vi "New motor Control integrated, NavX correction.vi"(1 "wTargetSpeed":dbl, 2 "yTargetSpeed":dbl, 3 "xTargetSpeed":dbl) -> (0 "Speed":T2)   [LabVIEW 2018]
panel:
  in  "Reset Encoder 0":bool
  in  "Boolean":bool=TRUE
  out "Distance":T1
  out "wSpeed":dbl
  out "ySpeed":dbl
  out "xSpeed":dbl
  out "Distance M2":dbl
  out "Distance M1":dbl
  out "Distance M0":dbl
  out "Motor Error":errorcluster
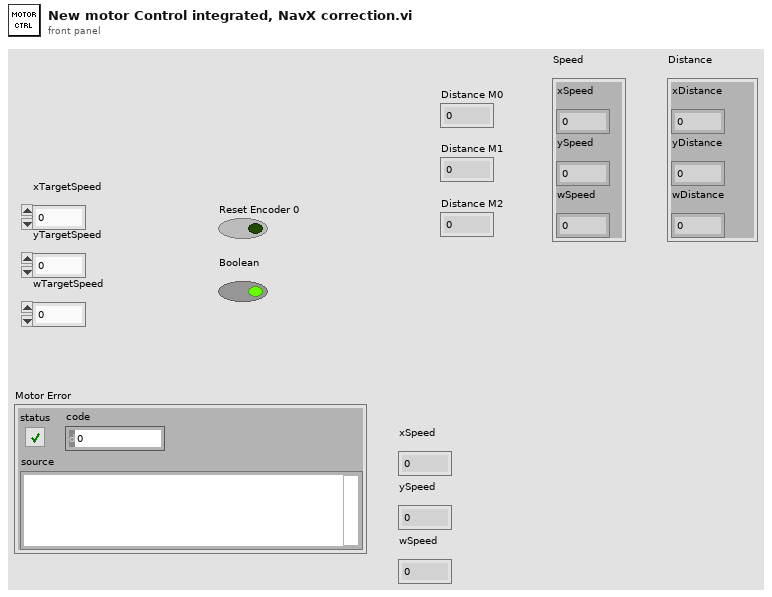
[diagram p1: front panel]
types:
  T1 = cluster{"xDistance":dbl, "yDistance":dbl, "wDistance":dbl}
  T2 = cluster{"xSpeed":dbl, "ySpeed":dbl, "wSpeed":dbl}
  T3 = cluster{"Encoder 0":dbl, "Encoder 1":dbl, "Encoder 2":dbl}
  T4 = cluster{"Distance M0 ":dbl, "Distance M1 ":dbl, "Distance M2 ":dbl}
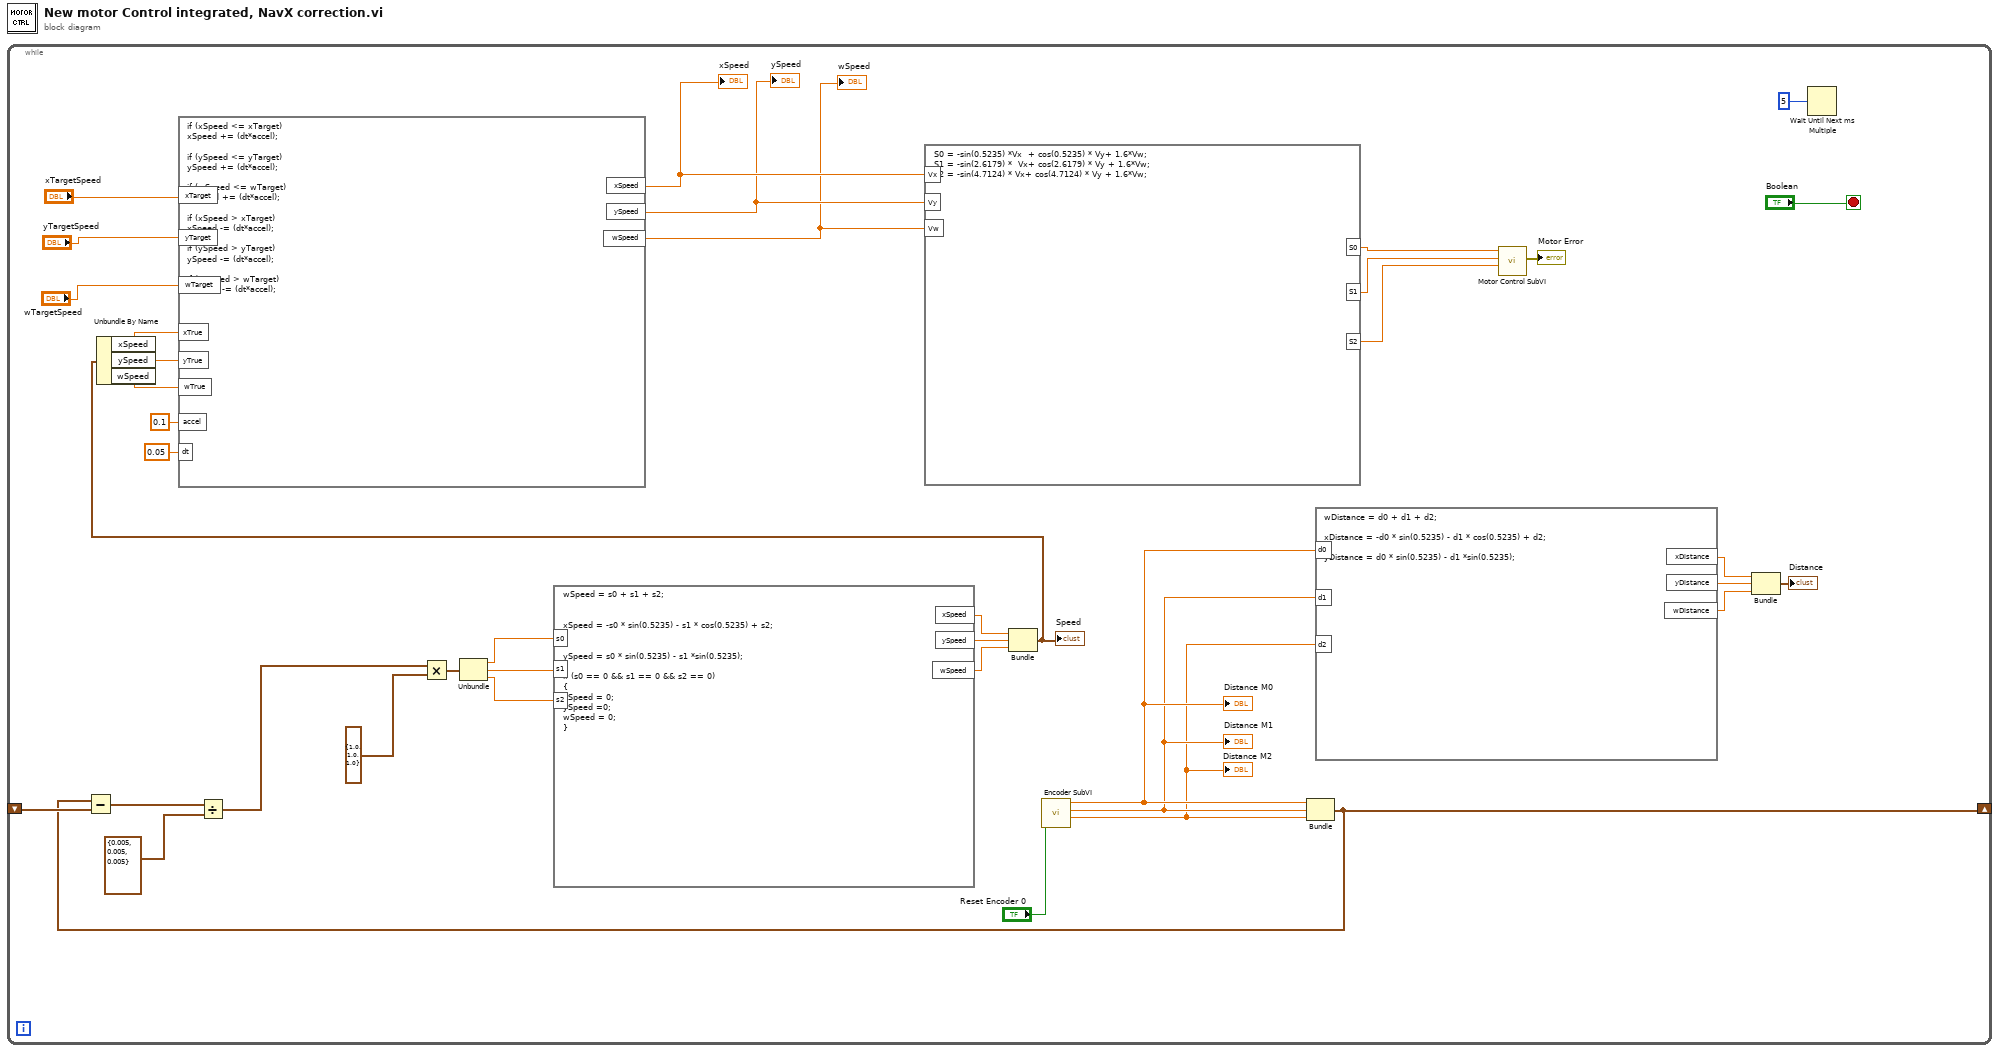
[diagram p0: block diagram]
diagram:
  n1 = while {
    shift-right: [w15] -> _
    shift-left: _ -> [w16]
    stop <- "Boolean" stop-if-true
    n2 = call "Encoder SubVI.vi"("Reset Encoders"="Reset Encoder 0") -> ("Distance M2"=w11:dbl, "Distance M1"=w12:dbl, "Distance M0"=w13:dbl)  [unwired: 7 in, 1 out]
    "Distance M0" <- w13
    "Distance M1" <- w12
    "Distance M2" <- w11
    n3 = Bundle("Distance M0"=w13, "Distance M1"=w12, "Distance M2"=w11) -> (w15:T4)  [unwired: 1 in]
    n4 = Subtract(x=w15, y=w16) -> (x-y=w38:T4)
    n5 = Divide(x=w38, y=T3 {"Encoder 0"=0.005, "Encoder 1"=0.005, "Encoder 2"=0.005}) -> (x/y=w5:cluster{dbl, dbl, dbl})
    n6 = Multiply(x=w5, y=cluster{dbl, dbl, dbl} {1.0, 1.0, 1.0}) -> (x*y=w3:cluster{dbl, dbl, dbl})
    n7 = Unbundle(w3) -> (w1:dbl, w26:dbl, w25:dbl)
    n8 = formula code="wSpeed = s0 + s1 + s2;\n\n\nxSpeed = -s0 * sin(0.5235) - s1 * cos(0.5235) + s2;\n\n\nySpeed = s0 * sin(0.5235) - s1 *sin(0.5235);\n\nif (s0 == 0 && s1 == 0 && s2 == 0)\n{\nxSpeed = 0;\nySpeed =0;\nwSpeed = 0;\n}"("s0"=w1, "s1"=w26, "s2"=w25) -> ("xSpeed"=w35:dbl, "ySpeed"=w36:dbl, "wSpeed"=w34:dbl)
    n9 = Bundle("xSpeed"=w35, "ySpeed"=w36, "wSpeed"=w34) -> (w33:T2)  [unwired: 1 in]
    "Speed" <- w33
    n10 = Unbundle By Name(w33) -> ("xSpeed"=w32:dbl, "ySpeed"=w31:dbl, "wSpeed"=w30:dbl)
    n11 = formula code="if (xSpeed <= xTarget)\nxSpeed += (dt*accel);\n\nif (ySpeed <= yTarget)\nySpeed += (dt*accel);\n\nif (wSpeed <= wTarget)\nwSpeed += (dt*accel);\n\nif (xSpeed > xTarget)\nxSpeed -= (dt*accel);\n\nif (ySpeed > yTarget)\nySpeed -= (dt*accel);\n\nif (wSpeed > wTarget)\nwSpeed -= (dt*accel);"("xTarget"="xTargetSpeed", "yTarget"="yTargetSpeed", "wTarget"="wTargetSpeed", "xTrue"=w32, "yTrue"=w31, "wTrue"=w30, "accel"=0.1 ("input variable"), "dt"=0.05 ("input variable")) -> ("xSpeed"=w24:dbl, "ySpeed"=w23:dbl, "wSpeed"=w22:dbl)
    "xSpeed" <- w24
    "ySpeed" <- w23
    "wSpeed" <- w22
    n12 = formula code="S0 = -sin(0.5235) *Vx  + cos(0.5235) * Vy+ 1.6*Vw;\nS1 = -sin(2.6179) *  Vx+ cos(2.6179) * Vy + 1.6*Vw;\nS2 = -sin(4.7124) * Vx+ cos(4.7124) * Vy + 1.6*Vw;"("Vx"=w24, "Vy"=w23, "Vw"=w22) -> ("S0"=w2:dbl, "S1"=w18:dbl, "S2"=w17:dbl)
    n13 = formula code="wDistance = d0 + d1 + d2;\n\nxDistance = -d0 * sin(0.5235) - d1 * cos(0.5235) + d2;\n\nyDistance = d0 * sin(0.5235) - d1 *sin(0.5235);"("d0"=w13, "d1"=w12, "d2"=w11) -> ("xDistance"=w10:dbl, "wDistance"=w8:dbl, "yDistance"=w9:dbl)
    n14 = call "Motor Control SubVI.vi"("Speed M2"=w17, "Speed M1"=w18, "Speed M0"=w2) -> ("Motor Error"=→"Motor Error":errorcluster)  [unwired: 8 in]
    n15 = Bundle("xDistance"=w10, "yDistance"=w9, "wDistance"=w8) -> (→"Distance":T1)  [unwired: 1 in]
    n16 = Wait Until Next ms Multiple(millisecond multiple=u32 5) -> ()  [unwired: 1 out]
  }
